vi "Get State.vi"(8 "error in":errorcluster, 11 "TDCManager":T1) -> (0 "error out":errorcluster, 1 "State string":string, 2 "State":i32, 3 "TDCManager":T1)   [LabVIEW 2016, in "HPTDC Driver Library.lvlib"]
uses:
  HPTDC Driver Library.lvlib
  Typedefs/TDCManager.ctl
  C:/Users/CRT Controller/CRTC Labview Application/Source/HPTDC Driver Library Folder/Library files/hptdc_net4_3.7.0_x64.dll
  hptdc_net4_3.7.0_x64.dll
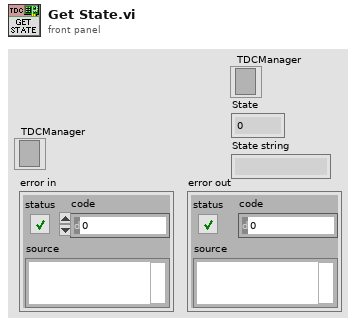
[diagram p1: front panel]
types:
  T1 = typedef "HPTDC Driver Library.lvlib/TDCManager.ctl" = refnum<k24>
  T2 = typedef "Semaphore RefNum" = refnum<k1>
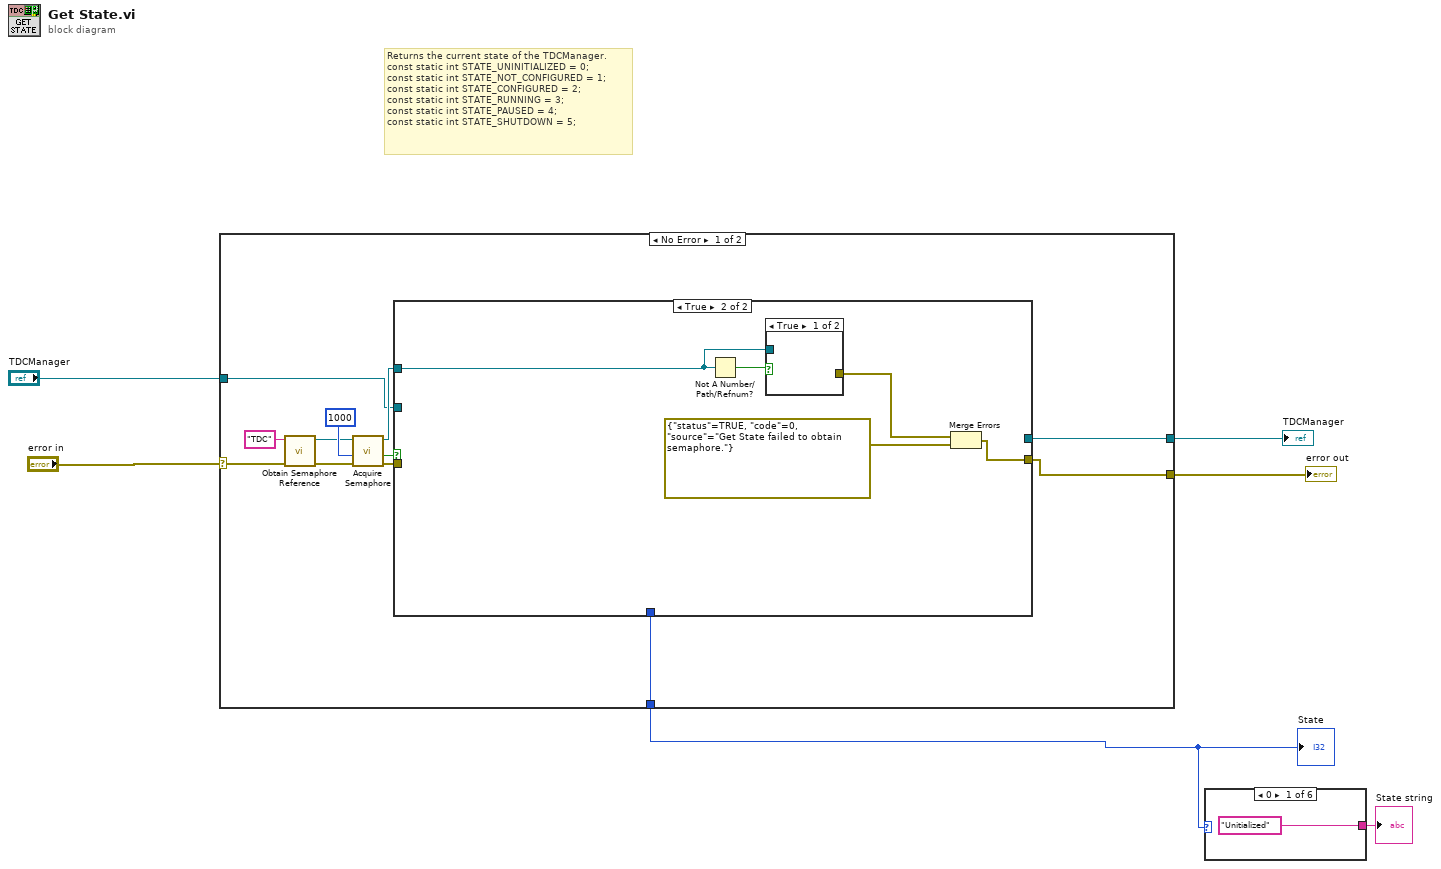
[diagram p0: block diagram]
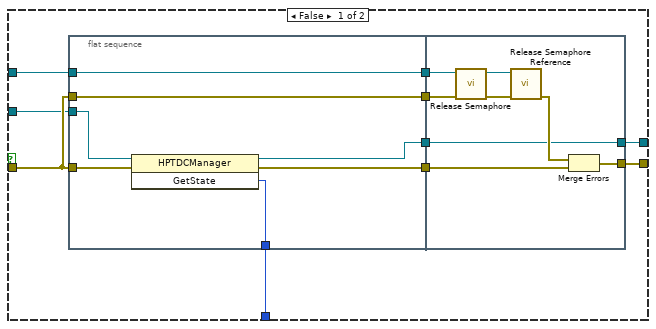
[diagram p2: hidden frame]
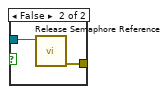
[diagram p3: hidden frame]
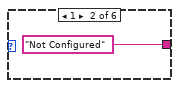
[diagram p5: hidden frame]
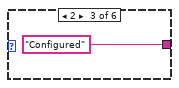
[diagram p6: hidden frame]
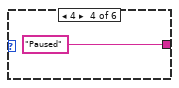
[diagram p7: hidden frame]
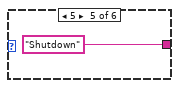
[diagram p8: hidden frame]
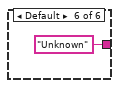
[diagram p9: hidden frame]
diagram:
  # "Returns the current state of the TDCManager.\nconst static int STATE_UNINITIALIZED = 0;\nconst static int STATE_NOT_CONFIGURED = 1;\nconst static int STATE_CONFIGURED = 2;\nconst static int STATE_RUNNING = 3;\nconst static int STATE_PAUSED = 4;\nconst static int STATE_SHUTDOWN = 5;"
  n1 = case shown="No Error" "error in" {
    selector: "error in" -> [w7 w52]
    tunnel: "TDCManager" -> [w13 w51]
    tunnel: [w12 w51] -> w4
    tunnel: [w11 _] -> w3
    tunnel: [w10 w52] -> w2
    frame No Error {
      n2 = call <vilib>:"Obtain Semaphore Reference.vi"("error in (no error)"=w7, "name (unnamed)"="TDC") -> ("error out"=w8:errorcluster, "semaphore"=w9:T2)  [unwired: 3 in, 1 out]
      n3 = call <vilib>:"Acquire Semaphore.vi"("error in (no error)"=w8, "ms timeout (-1)"=1000, "semaphore"=w9) -> ("error out"=w15:errorcluster, "timed out"=w16:bool, "semaphore out"=w14:T2)  [unwired: 2 in]
      n4 = case shown="True" w16 {
        tunnel: w15 -> [w26 _]
        tunnel: w14 -> [w24 w44]
        tunnel: [w21 _] -> w12
        tunnel: [w23 w46] -> w10
        tunnel: w13 -> [w20 _]
        tunnel: [w19 _] -> w11
        frame False {
          n5 = flat-sequence {
            tunnel: w26 -> [w31]
            tunnel: [w33] -> w28
            tunnel: w26 -> [w35]
            tunnel: [w35] -> w27
            tunnel: [w34] -> w25
            tunnel: w24 -> [w34]
            tunnel: [w32] -> w22
            tunnel: w20 -> [w30]
            tunnel: [w29] -> w19
            tunnel: w28 -> [w43]
            tunnel: w27 -> [w40]
            tunnel: w25 -> [w38]
            tunnel: [w37] -> w23
            tunnel: [w36] -> w21
            tunnel: w22 -> [w36]
            frame #0 {
              n6 = invoke class="HPTDCManager" method="GetState"(reference=w30, error in=w31) -> (reference out=w32:T1, error out=w33:errorcluster, "GetState"=w29:i32)  [unwired: 1 in]
            }
            frame #1 {
              n7 = call <vilib>:"Release Semaphore.vi"("error in (no error)"=w40, "semaphore"=w38) -> ("error out"=w41:errorcluster, "semaphore out"=w42:T2)  [unwired: 4 in]
              n8 = call <vilib>:"Release Semaphore Reference.vi"("error in (no error)"=w41, "semaphore"=w42) -> ("error out"=w39:errorcluster)  [unwired: 8 in, 1 out]
              n9 = Merge Errors(w39, w43) -> (w37:errorcluster)
            }
          }
        }
        frame True {
          n10 = Not A Number/Path/Refnum?(number/path/refnum=w44) -> (NaN/Path/Refnum?=w48:bool)
          n11 = case shown="True" w48 {
            tunnel: [_ w50] -> w45
            tunnel: w44 -> [_ w49]
            frame True {
            }
            frame False {
              n12 = call <vilib>:"Release Semaphore Reference.vi"("semaphore"=w49) -> ("error out"=w50:errorcluster)  [unwired: 9 in, 1 out]
            }
          }
          n13 = Merge Errors(w45, errorcluster {"status"=TRUE, "code"=0, "source"="Get State failed to obtain semaphore."} ("error out")) -> (w46:errorcluster)
        }
      }
    }
    frame Error {
    }
  }
  "TDCManager" <- w4
  "State" <- w3
  "error out" <- w2
  n14 = case shown="0" w3 {
    tunnel: ["Unitialized" "Not Configured" "Configured" "Paused" "Shutdown" "Unknown"] -> w6
    frame 0 {
    }
    frame 1 {
    }
    frame 2 {
    }
    frame 4 {
    }
    frame 5 {
    }
    frame Default {
    }
  }
  "State string" <- w6
